vi "Camera xyhl 1P.vi"(10 "tableau":u8[](array[numeric])) -> (2 "Indications pokaenmon":T1)   [LabVIEW 2013]
panel:
  out "sign":string
  out "h":string
  out "L":string
  out "y":string
  out "x":string
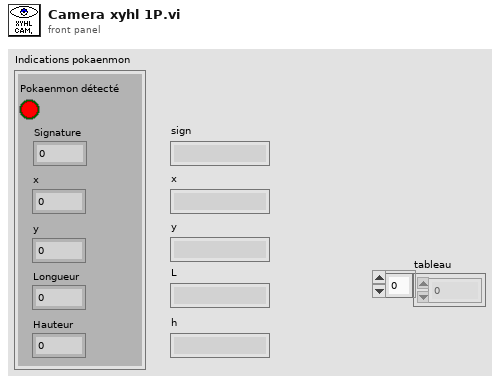
[diagram p1: front panel]
types:
  T1 = cluster{"Pokaenmon détecté":bool, "Signature":u32, "x":dbl, "y ":dbl, "Longueur":dbl, "Hauteur":dbl}
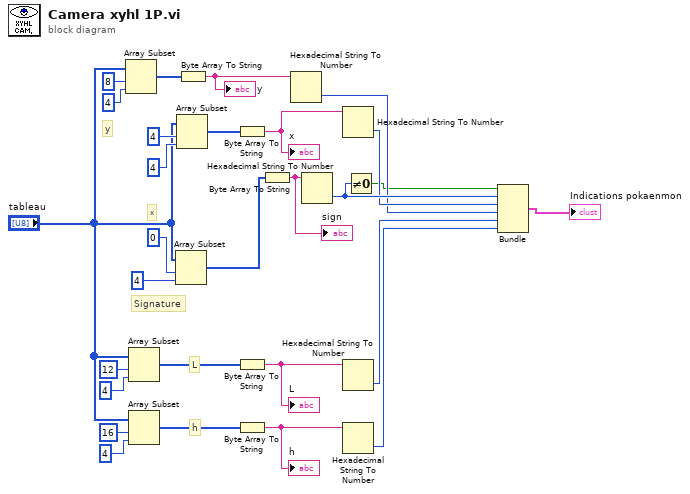
[diagram p0: block diagram]
diagram:
  # "h"
  # "L"
  # "y"
  # "x"
  # "Signature"
  n1 = Array Subset(array="tableau", index=8 ("offset (0)"), length=4 ("longueur (reste)")) -> (w15:u8[])
  n2 = Array Subset(array="tableau", index=12 ("offset (0)"), length=4 ("longueur (reste)")) -> (w16:u8[])
  n3 = Array Subset(array="tableau", index=16 ("offset (0)"), length=4 ("longueur (reste)")) -> (w17:u8[])
  n4 = Array Subset(array="tableau", index=0 ("offset (0)"), length=4 ("longueur (reste)")) -> (w27:u8[])
  n5 = Array Subset(array="tableau", index=4 ("offset (0)"), length=4 ("longueur (reste)")) -> (w14:u8[])
  n6 = Byte Array To String(unsigned byte array=w15) -> (string=w20:string)
  "y" <- w20
  n7 = Byte Array To String(unsigned byte array=w14) -> (string=w22:string)
  "x" <- w22
  n8 = Byte Array To String(unsigned byte array=w16) -> (string=w19:string)
  "L" <- w19
  n9 = Byte Array To String(unsigned byte array=w17) -> (string=w24:string)
  "h" <- w24
  n10 = Byte Array To String(unsigned byte array=w27) -> (string=w28:string)
  "sign" <- w28
  n11 = Hexadecimal String To Number(string=w20) -> (number=w21:u32)  [unwired: 2 in, 1 out]
  n12 = Hexadecimal String To Number(string=w28) -> (number=w26:u32)  [unwired: 2 in, 1 out]
  n13 = Hexadecimal String To Number(string=w22) -> (number=w23:u32)  [unwired: 2 in, 1 out]
  n14 = Hexadecimal String To Number(string=w19) -> (number=w18:u32)  [unwired: 2 in, 1 out]
  n15 = Hexadecimal String To Number(string=w24) -> (number=w25:u32)  [unwired: 2 in, 1 out]
  n16 = Not Equal To 0?(x=w26) -> (x != 0?=w3:bool)
  n17 = Bundle(w3, w26, w23, w21, w18, w25) -> (→"Indications pokaenmon":cluster{bool, u32, u32, u32, u32, u32})  [unwired: 1 in]
